vi "Vision Processing.vi"(4 "error in (no error)":errorcluster, 7 "Image Size":T1=enum."320x240") -> ()   [LabVIEW 2013]
doc: "This VI runs in parallel to other tasks. It gets images from the camera, processes them for color or shape and use that information to affect robot behavior."
uses:
  <vilib>/Rock Robotics/WPI/Camera/WPI_CameraImageSize.ctl
  <vilib>/Rock Robotics/WPI/Camera/WPI_CameraWhite Balance Values.ctl
  <vilib>/Rock Robotics/WPI/Camera/WPI_CameraExposure Values.ctl
  <vilib>/Rock Robotics/WPI/Camera/WPI_CameraFrameRate.ctl
  2014 Robot Project 2-11-14/Robot Global Data.vi
  Robot Global Var.vi
panel:
  in  "Reliable?":bool=TRUE
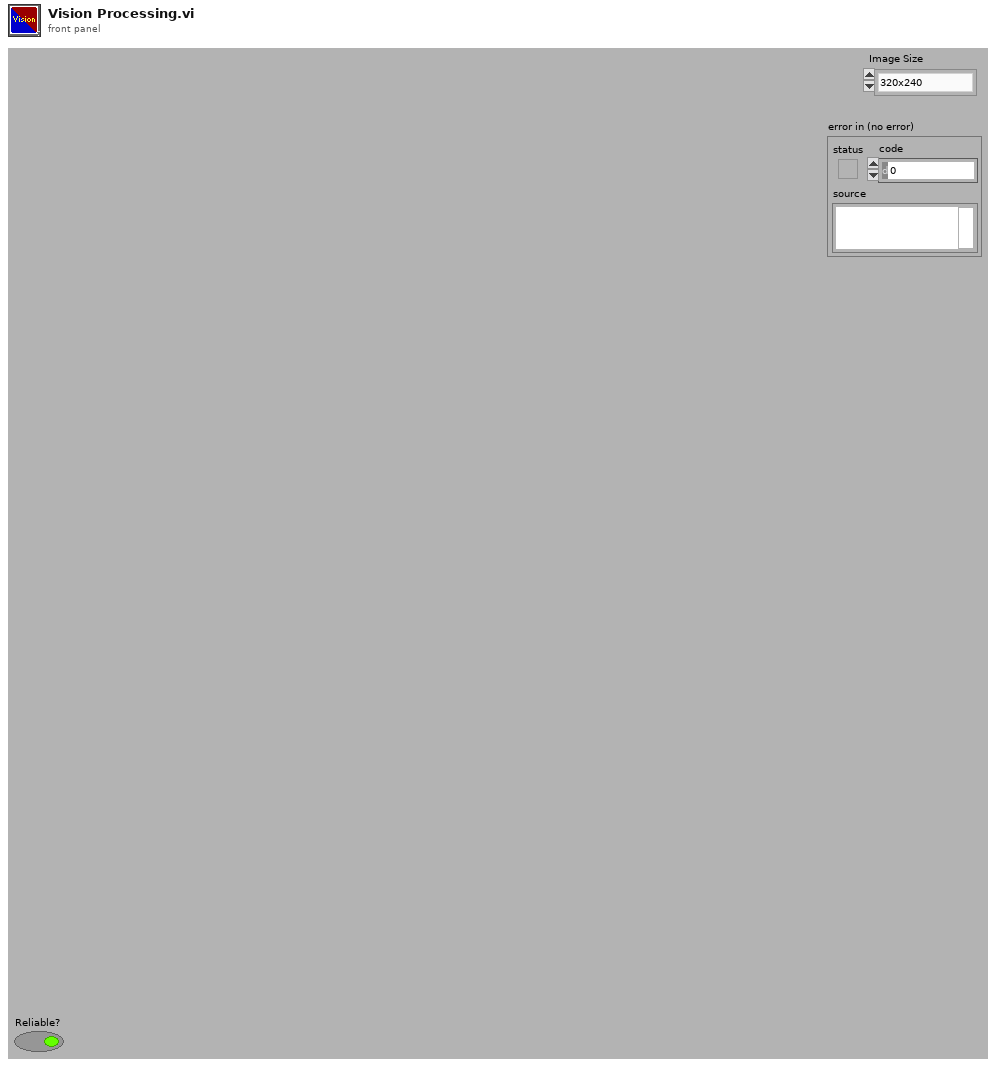
[diagram p1: front panel]
types:
  T1 = typedef "WPI_CameraImageSize.ctl" = enum16{"640x480", "320x240", "160x120"}
  T2 = typedef "WPI_CameraFrameRate.ctl" = u32
  T3 = typedef "WPI_CameraExposure Values.ctl" = enum16{"Auto", "Flicker-free 50 Hz", "Flicker-free 60 Hz", "Hold current"}
  T4 = typedef "WPI_CameraWhite Balance Values.ctl" = enum16{"Auto", "Fixed indoor", "Fixed outdoor 1", "Fixed outdoor 2", "Fixed fluorescent 1", "Fixed fluorescent 2", "Hold current"}
  T5 = typedef "Image Type" = u32
  T6 = typedef "WPI_CameraDevRef.ctl" = cluster{"Camera Address":string, "CameraStatus":errorcluster, "Acquire Image Notifier":refnum<notifier>}
  T7 = typedef "IMAQ Image.ctl" = refnum<image>
  T8 = typedef "WPI_DriverStationRobotMode2.ctl" = enum16{"Autonomous Disabled", "Autonomous Enabled", "Teleop Disabled", "Teleop Enabled", "Timeout", "Finish", "Test Disabled", "Test Enabled"}
  T9 = cluster{cluster{"Numeric":dbl, "Numeric":dbl}, cluster{"Numeric":dbl, "Numeric":dbl}, cluster{"Numeric":dbl, "Numeric":dbl}}
  T10 = cluster{"Horizontal":bool, "Aspect Score":dbl, "Rect Score":dbl, cluster{"Left":dbl, "Top":dbl, "Right":dbl, "Bottom":dbl}, "Equiv H":dbl, "Equiv V":dbl}[]
  T11 = typedef "TargetType.ctl" = enum16{"Not Hot", "Hot"}
  T12 = cluster{"Scores":cluster{"Total":dbl, "Left":dbl, "Right":dbl, "Ratio":dbl, "Vertical":dbl, "index":i32, "State":T11}, "Verticals":cluster{"Horizontal?":bool, "Aspect Score":dbl, "Rect Score":dbl, cluster{"Left":dbl, "Top":dbl, "Right":dbl, "Bottom":dbl}, "Equiv H":dbl, "Equiv V":dbl}, "Horizontals":cluster{"Horizontal?":bool, "Aspect Score":dbl, "Rect Score":dbl, cluster{"Left":dbl, "Top":dbl, "Right":dbl, "Bottom":dbl}, "Equiv H":dbl, "Equiv V":dbl}, "Validated":bool}[]
  T13 = cluster{"Scores":cluster{"Total":dbl, "Left":dbl, "Right":dbl, "Ratio":dbl, "Vertical":dbl, "index":i32, "State":T11}, "Verticals":cluster{"Horizontal?":bool, "Aspect Score":dbl, "Rect Score":dbl, cluster{"Left":dbl, "Top":dbl, "Right":dbl, "Bottom":dbl}, "Equiv H":dbl, "Equiv V":dbl}, "Horizontals":cluster{"Horizontal?":bool, "Aspect Score":dbl, "Rect Score":dbl, cluster{"Left":dbl, "Top":dbl, "Right":dbl, "Bottom":dbl}, "Equiv H":dbl, "Equiv V":dbl}, "Distance (ft)":dbl, "Target Center (-1 to 1)":cluster{"X":dbl, "Y":dbl}}[]
  T14 = cluster{"Scores":cluster{"Total":dbl, "Left":dbl, "Right":dbl, "Ratio":dbl, "Vertical":dbl, "index":i32, "State":T11}, "Verticals":cluster{"Horizontal?":bool, "Aspect Score":dbl, "Rect Score":dbl, cluster{"Left":dbl, "Top":dbl, "Right":dbl, "Bottom":dbl}, "Equiv H":dbl, "Equiv V":dbl}, "Horizontals":cluster{"Horizontal?":bool, "Aspect Score":dbl, "Rect Score":dbl, cluster{"Left":dbl, "Top":dbl, "Right":dbl, "Bottom":dbl}, "Equiv H":dbl, "Equiv V":dbl}, "Distance (ft)":dbl, "Target Center (-1 to 1)":cluster{"X":dbl, "Y":dbl}}
  T15 = cluster{"Total":dbl, "Left":dbl, "Right":dbl, "Ratio":dbl, "Vertical":dbl, "index":i32, "State":T11}
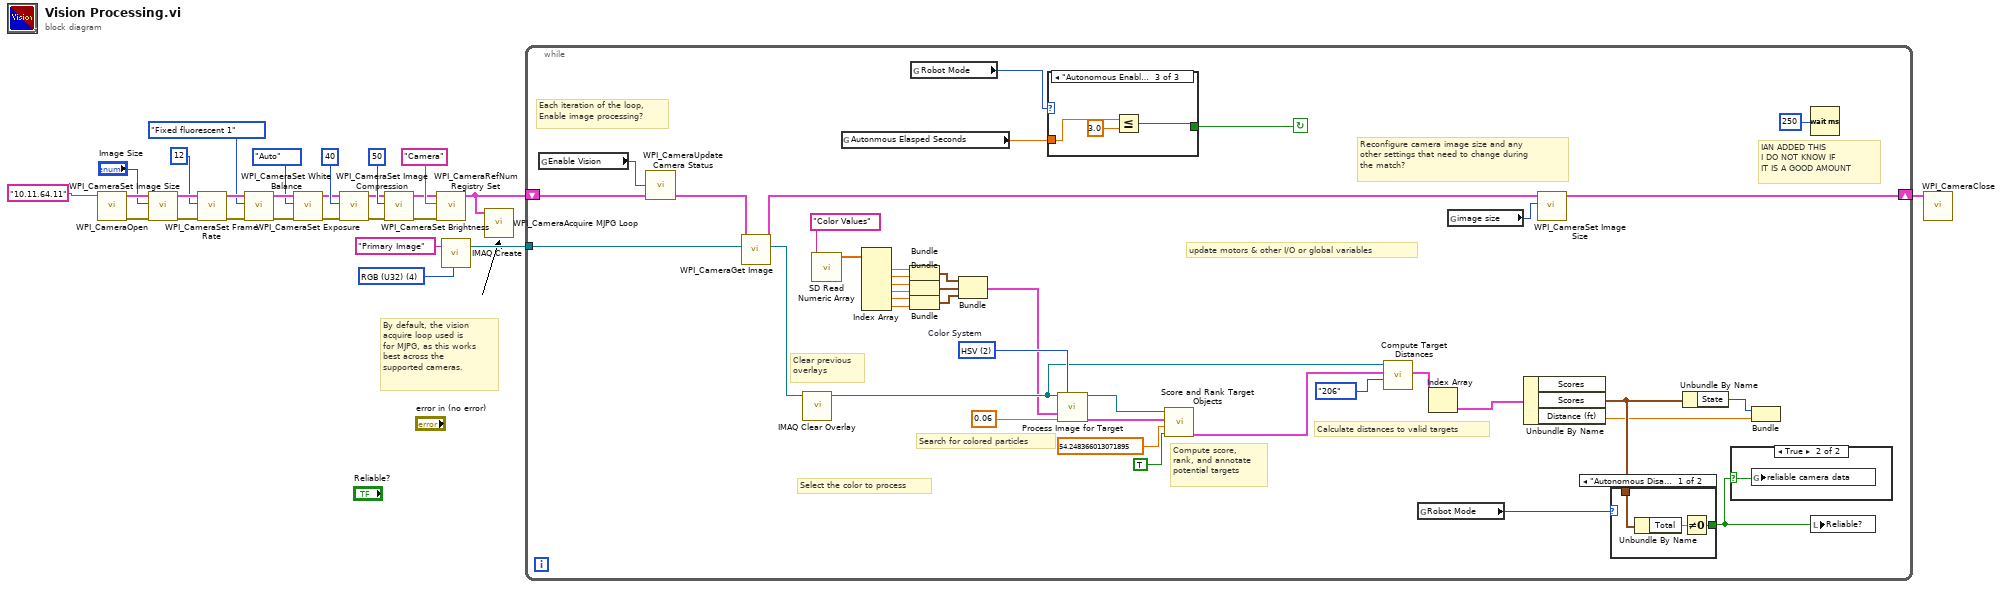
[diagram p0: block diagram]
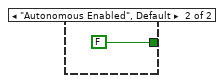
[diagram p3: hidden frame]
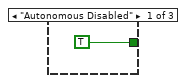
[diagram p4: hidden frame]
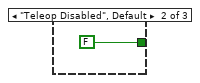
[diagram p5: hidden frame]
diagram:
  w27 = T5 4 items=["Grayscale (U8)", "Grayscale (I16)", "Grayscale (SGL)", "Complex (CSG)", "RGB (U32)", "HSL (U32)", "RGB (U64)"] ("Image Type")
  # "By default, the vision\nacquire loop used is\nfor MJPG, as this works\nbest across the\nsupported cameras."
  n1 = call <vilib>:"WPI_CameraOpen.vi"("Camera Address"="10.11.64.11" ("format string")) -> ("error out"=w15:errorcluster, "CameraDevRef"=w16:T6)  [unwired: 1 in, 8 out]
  n2 = call <vilib>:"WPI_CameraSet Image Size.vi"("error in (no error)"=w15, "Image Size"="Image Size", "CameraDevRef"=w16) -> ("error out"=w14:errorcluster, "CameraDevRef Out"=w17:T6)  [unwired: 7 out]
  n3 = call <vilib>:"WPI_CameraSet Frame Rate.vi"("error in (no error)"=w14, "Frame Rate (fps)"=T2 12, "CameraDevRef"=w17) -> ("error out"=w13:errorcluster, "CameraDevRef Out"=w19:T6)  [unwired: 7 out]
  n4 = call <vilib>:"WPI_CameraSet White Balance.vi"("error in (no error)"=w13, "White Balance"=WPI_CameraWhite_Balance_Values."Fixed fluorescent 1", "CameraDevRef"=w19) -> ("error out"=w12:errorcluster, "CameraDevRef Out"=w18:T6)  [unwired: 7 out]
  n5 = call <vilib>:"WPI_CameraSet Exposure.vi"("error in (no error)"=w12, "Exposure"=WPI_CameraExposure_Values."Auto", "CameraDevRef"=w18) -> ("error out"=w11:errorcluster, "CameraDevRef Out"=w21:T6)  [unwired: 7 out]
  n6 = call <vilib>:"WPI_CameraSet Image Compression.vi"("error in (no error)"=w11, "Compression"=40, "CameraDevRef"=w21) -> ("error out"=w10:errorcluster, "CameraDevRef Out"=w20:T6)  [unwired: 7 out]
  n7 = call <vilib>:"WPI_CameraSet Brightness.vi"("error in (no error)"=w10, "Brightness"=50, "CameraDevRef"=w20) -> ("error out"=w8:errorcluster, "CameraDevRef Out"=w9:T6)  [unwired: 7 out]
  n8 = call <vilib>:"WPI_CameraRefNum Registry Set.vi"("error in (no error)"=w8, "refnum name"="Camera", "CameraDevRef"=w9) -> ("CameraDevRef"=w4:T6)  [unwired: 8 out]
  n9 = call "IMAQ Create"("Image Name"="Primary Image", "Image Type"=w27) -> ("New Image"=w25:T7)  [unwired: 2 in, 2 out]
  n10 = call <vilib>:"WPI_CameraAcquire MJPG Loop.vi"("CameraDevRef"=w4) -> ()  [unwired: 11 in]
  n11 = while {
    tunnel: w25 -> [w67]
    shift-right: [w47] -> w1
    shift-left: w4 -> [w66]
    stop <- w48 continue-if-true
    w55 = u16 2 items=["RGB", "HSL", "HSV", "HSI"]  # Color System
    # "IAN ADDED THIS\nI DO NOT KNOW IF\nIT IS A GOOD AMOUNT"
    # "Clear previous\noverlays"
    # "Calculate distances to valid targets"
    # "Search for colored particles"
    # "Compute score,\nrank, and annotate\npotential targets"
    # "Select the color to process"
    # "update motors & other I/O or global variables"
    # "Reconfigure camera image size and any\nother settings that need to change during\nthe match?"
    # "Each iteration of the loop,\nEnable image processing?"
    n12 = global read "Robot Global Data.vi" "Enable Vision"() -> (w64:bool)
    n13 = call <vilib>:"WPI_CameraUpdate Camera Status.vi"("CameraDevRef In"=w66, "Enable Vision"=w64) -> ("CameraDevRef Out"=w65:T6)  [unwired: 3 in]
    n14 = call <vilib>:"WPI_CameraGet Image.vi"("Image"=w67, "CameraDevRef"=w65) -> ("Image Out"=w52:T7, "CameraDevRef Out"=w62:T6)  [unwired: 1 in, 7 out]
    n15 = call "IMAQ Clear Overlay"("Image"=w52) -> ("Image Out"=w54:T7)  [unwired: 9 in, 1 out]
    n16 = call <vilib>:"SD Read Numeric Array.vi"("Name"="Color Values") -> ("Numeric Array"=w44:dbl[])  [unwired: 8 in, 2 out]
    n17 = global read "Robot Global Var.vi" "Autonmous Elasped Seconds"() -> (w28:dbl)
    n18 = Index Array(array=w44) -> (element #1=w42:dbl, element #2=w43:dbl, element #3=w41:dbl, element #4=w40:dbl, element #5=w39:dbl, element #6=w38:dbl)  [unwired: 6 in]
    n19 = Bundle("Numeric"=w42, "Numeric"=w43) -> (w37:cluster{"Numeric":dbl, "Numeric":dbl})  [unwired: 1 in]
    n20 = Bundle("Numeric"=w41, "Numeric"=w40) -> (w36:cluster{"Numeric":dbl, "Numeric":dbl})  [unwired: 1 in]
    n21 = Bundle("Numeric"=w39, "Numeric"=w38) -> (w35:cluster{"Numeric":dbl, "Numeric":dbl})  [unwired: 1 in]
    n22 = global read "Robot Global Data.vi" "Robot Mode"() -> (w49:T8)
    n23 = Bundle(w37, w36, w35) -> (w34:T9)  [unwired: 1 in]
    n24 = case shown="\"Autonomous Enabled\"" w49 {
      tunnel: [TRUE FALSE w77] -> w48
      tunnel: w28 -> [_ _ w75]
      frame "Autonomous Disabled" {
      }
      frame "Teleop Disabled", Default {
      }
      frame "Autonomous Enabled" {
        n25 = Less Or Equal?(x=w75, y=3.0) -> (x <= y?=w77:bool)
      }
    }
    n26 = call "Process Image for Target.vi"("Src Image"=w54, "Color Mode"=w55, "Color Components"=w34, "Area Cutoff %"=0.06 ("Area Size Limit %")) -> ("Src Image Out"=w60:T7, "Particles"=w58:T10)  [unwired: 9 in, 1 out]
    n27 = call "Score and Rank Target Objects.vi"("Annotate"=TRUE, "Score Limit"=54.248366013071895 ("Score Cutoff"), "Particles"=w58, "Image in"=w60) -> ("Target Info"=w57:T12)  [unwired: 6 in, 1 out]
    n28 = call "Compute Target Distances.vi"("Camera Type"=enum16{"206", "1011", "1013"}."206", "Target Info"=w57, "Image in"=w54) -> ("Target Info"=w51:T13)  [unwired: 6 in, 2 out]
    n29 = global read "Robot Global Data.vi" "Robot Mode"() -> (w46:T8)
    n30 = Index Array(array=w51) -> (element=w50:T14)  [unwired: 1 in]
    n31 = global read "Robot Global Data.vi" "image size"() -> (w63:T1)
    n32 = Unbundle By Name(w50) -> ("Scores"=w45:T15, "Distance (ft)"=w31:dbl)  [unwired: 1 out]
    n33 = call <vilib>:"WPI_CameraSet Image Size.vi"("Image Size"=w63, "CameraDevRef"=w62) -> ("CameraDevRef Out"=w47:T6)  [unwired: 1 in, 8 out]
    n34 = case shown="\"Autonomous Disabled\"" w46 {
      tunnel: w45 -> [w71 _]
      tunnel: [w69 FALSE ("Reliable? 2")] -> w29
      frame "Autonomous Disabled" {
        n35 = Unbundle By Name(w71) -> ("Total"=w70:dbl)
        n36 = Not Equal To 0?(x=w70) -> (x != 0?=w69:bool)
      }
      frame "Autonomous Enabled", Default {
      }
    }
    n37 = Unbundle By Name(w45) -> ("State"=w32:T11)
    n38 = case shown="True" w29 {
      selector: w29 -> [_ w68]
      frame False {
      }
      frame True {
        n39 = global write "Robot Global Var.vi" "reliable camera data"(w68) -> ()
      }
    }
    n40 = Bundle("State"=w32, "Distance (ft)"=w31) -> ()  [unwired: 1 in, 1 out]
    n41 = Wait (ms)(milliseconds to wait=u32 250) -> ()  [unwired: 1 out]
    n42 = local write "Reliable?"(w29) -> ()
  }
  n43 = call <vilib>:"WPI_CameraClose.vi"("CameraDevRef"=w1) -> ()  [unwired: 1 in, 10 out]
